vi "Write Force Sensor Calculator.vi"(10 "Force Sensor Calculator":T1={"Capacity"=1.0, "Sensitivity"=0.001, "Bridge Resistors"={"R1"=1.0, "R2"=1.0}} {"Bridge Resistors"."R2" min=1.0 max=5000000.0 format="%.1f"; "Bridge Resistors"."R1" min=1.0 max=5000000.0 format="%.1f"; "Sensitivity" min=0.001 max=5000.0 format="%.5f"; "Capacity" min=1.0 max=5000000.0 format="%.4f"}, 11 "ForceSensorCalculator in":refnum<class "ForceSensorCalculator.lvclass">) -> (3 "ForceSensorCalculator out":refnum<class "ForceSensorCalculator.lvclass">)   [LabVIEW 2013, in "ForceSensorCalculator.lvlib" / "ForceSensorCalculator.lvclass"]
uses:
  <userlib>/Common/Devices/ForceSensorCalculator/ForceSensorCalculator/ForceSensorCalculator.lvclass
  <userlib>/Common/Devices/ForceSensorCalculator/Config/Force Sensor Calculator.ctl
  <userlib>/Common/Devices/ForceSensorCalculator/Config/Bridge Resistors.ctl
  <userlib>/Common/Devices/ForceSensorCalculator/ForceSensorCalculator/ForceSensorCalculator.lvclass/ForceSensorCalculator.ctl
  <userlib>/Common/Devices/ForceSensorCalculator/ForceSensorCalculator.lvlib
panel:
  # "defined at capacity"
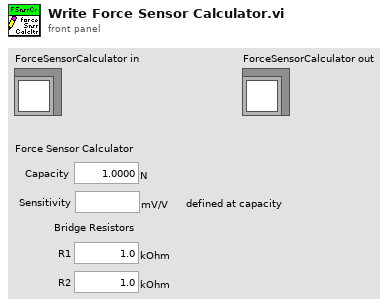
[diagram p1: front panel]
types:
  T1 = typedef "ForceSensorCalculator.lvlib/Force Sensor Calculator.ctl" = cluster{"Capacity":dbl[unit], "Sensitivity":dbl[unit], "Bridge Resistors":T2}
  T2 = typedef "ForceSensorCalculator.lvlib/Bridge Resistors.ctl" = cluster{"R1":dbl[unit], "R2":dbl[unit]}
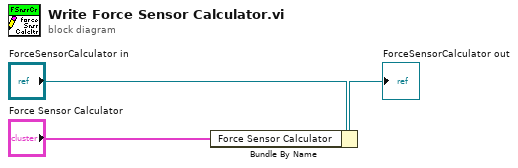
[diagram p0: block diagram]
diagram:
  n1 = Bundle By Name(cluster="ForceSensorCalculator in", "Force Sensor Calculator"="Force Sensor Calculator") -> (→"ForceSensorCalculator out":refnum<class "ForceSensorCalculator.lvclass">)
